vi "Set Block Size.vi"(8 "error in":errorcluster, 10 "Block Size":u8=16, 11 "Block Upload Initiate in":refnum<class "Block Upload Initiate Transfer.lvclass">) -> (0 "error out":errorcluster, 3 "Block Upload Initiate out":refnum<class "Block Upload Initiate Transfer.lvclass">)   [LabVIEW 2020, in "CANopen.lvlib" / "SDO Manager.lvlib" / "Block Upload Initiate Transfer.lvclass"]
uses:
  Block Upload Initiate Transfer.lvclass
  Block Upload Initiate Transfer.lvclass/Block Upload Initiate Transfer.ctl
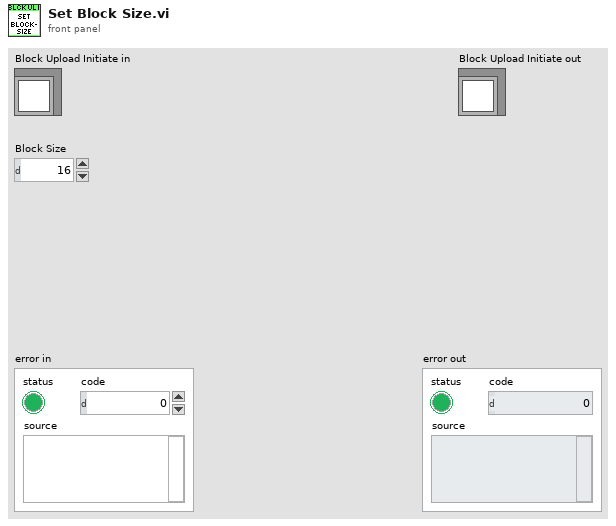
[diagram p1: front panel]
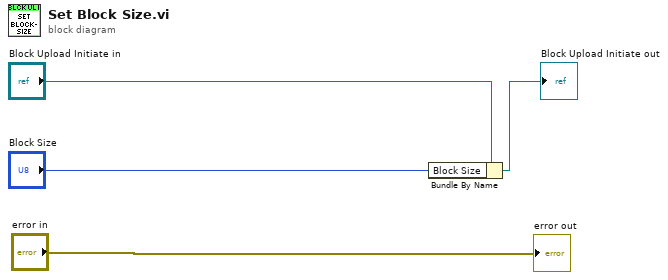
[diagram p0: block diagram]
diagram:
  n1 = Bundle By Name(cluster="Block Upload Initiate in", "Block Size"="Block Size") -> (→"Block Upload Initiate out":refnum<class "Block Upload Initiate Transfer.lvclass">)
  "error out" <- "error in"
